vi "u64.le.vi"(8 "end":u8=14, 9 "start":u8=6, 10 "Data":u8, 11 "Counter":u8) -> (3 "Latched\nValue":u64)   [LabVIEW 2022 SP3]
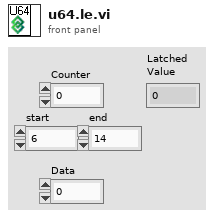
[diagram p1: front panel]
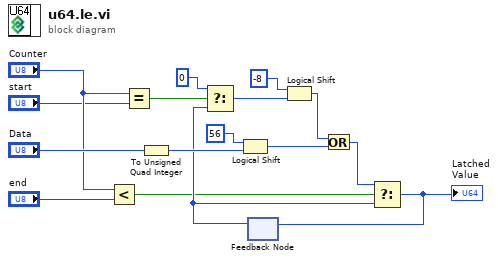
[diagram p0: block diagram]
diagram:
  n1 = Less?(x="Counter", y="end") -> (x < y?=w5:bool)
  n2 = Equal?(x="Counter", y="start") -> (x = y?=w3:bool)
  n3 = To Unsigned Quad Integer(1:"Data") -> (0:w10:u64)
  n4 = Logical Shift(y=i16 56, x=w10) -> (x << y=w11:u64)
  n5 = feedback #1() -> (w8:u64)  [unwired: 1 in]
  n6 = Select(t=u64 0 ("y"), s=w3, f=w8) -> (s? t:f=w12:u64)
  n7 = Logical Shift(y=i16 -8, x=w12) -> (x << y=w15:u64)
  n8 = Or(x=w15, y=w11) -> (x .or. y?=w13:u64)
  n9 = Select(t=w13, s=w5, f=w8) -> (s? t:f=w14:u64)
  "Latched\nValue" <- w14
  n10 = feedback-in #1(w14) -> ()
